vi "ESP301_Wait.vi"(10 "axisNumber":i32=1, 11 "COM_PORT":string="COM12") -> ()   [LabVIEW 2019]
uses:
  Newport.ESP301.CommandInterface
panel:
  out "errstring":string
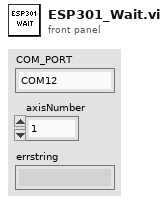
[diagram p1: front panel]
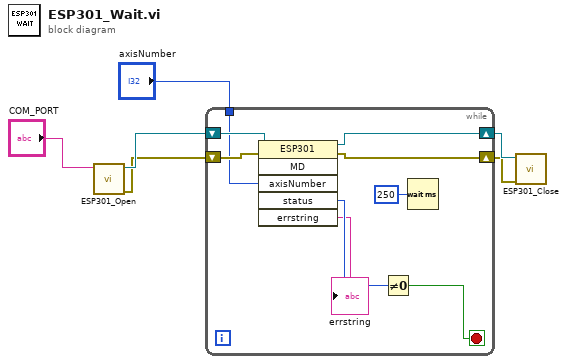
[diagram p0: block diagram]
diagram:
  n1 = call "ESP301_Open.vi"("strDeviceKey"="COM_PORT") -> ("sortie d'erreur"=w5:errorcluster, "référence en sortie"=w6:refnum<k24>)  [unwired: 9 in]
  n2 = while {
    tunnel: "axisNumber" -> [w13]
    shift-right: [w12] -> w2
    shift-left: w6 -> [w15]
    shift-right: [w11] -> w1
    shift-left: w5 -> [w14]
    stop <- w10 stop-if-true
    n3 = invoke on="Nœud de méthode" class="ESP301" method="MD"(reference=w15, error in=w14, "axisNumber"=w13) -> (reference out=w12:refnum<k24>, error out=w11:errorcluster, "status"=w9:i32, "errstring"=→"errstring":string)  [unwired: 3 in, 2 out]
    n4 = Not Equal To 0?(x=w9) -> (x != 0?=w10:bool)
    n5 = Wait (ms)(milliseconds to wait=u32 250 ("attente (ms)")) -> ()  [unwired: 1 out]
  }
  n6 = call "ESP301_Close.vi"("entrée d'erreur (pas d'erreur)"=w1, "référence"=w2) -> ()  [unwired: 9 in, 1 out]
